vi "Connection Alive FGV A.vi"(0 "command":T2, 1 "IP address":string, 5 "connection ID":refnum<k5>, 9 "Name":string, 11 "error in (no error)":errorcluster, 12 "Message":string) -> (3 "Messages":string[](array[string]), 4 "Cluster":T1, 6 "Variant Out":variant, 8 "All connections":T1[](array[typedef]), 10 "all connections":refnum<k5>[](array[refnum]), 13 "Names":string[](array[string]), 14 "IP Addresses":string[](array[string]), 15 "error out":errorcluster)   [LabVIEW 2020]
uses:
  Connection Info.ctl
  Command.ctl
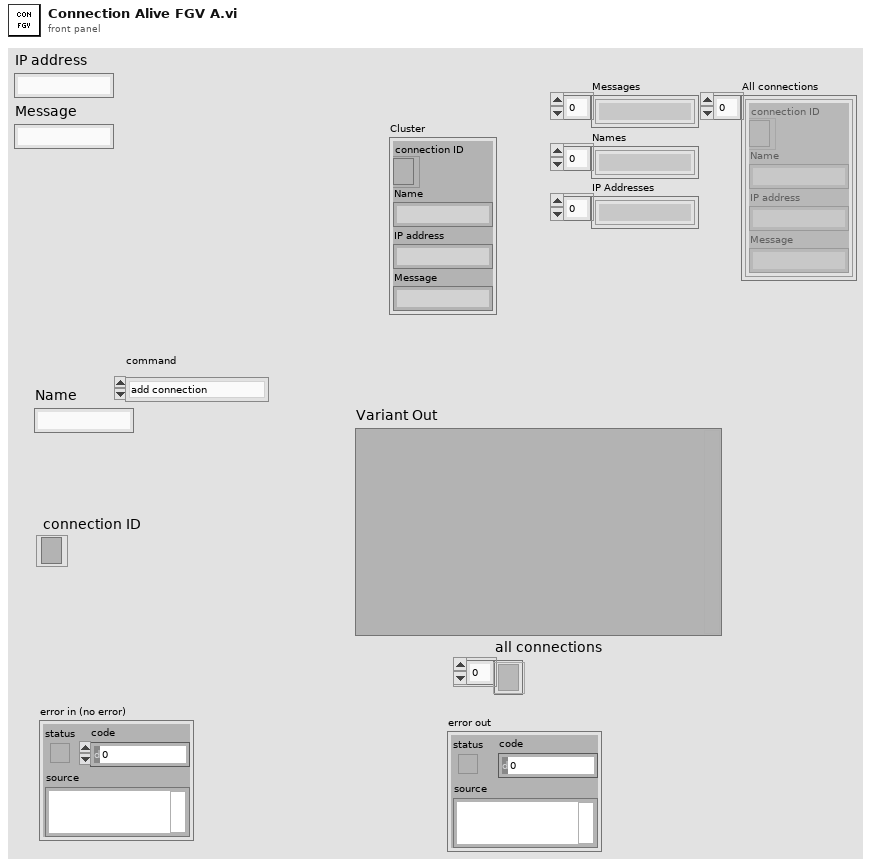
[diagram p1: front panel]
types:
  T1 = typedef "Connection Info.ctl" = cluster{"connection ID":refnum<k5>, "Name":string, "IP address":string, "Message":string}
  T2 = typedef "Command.ctl" = enum16{"add connection", "remove connection", "read connection data", "return all connections", "reset"}
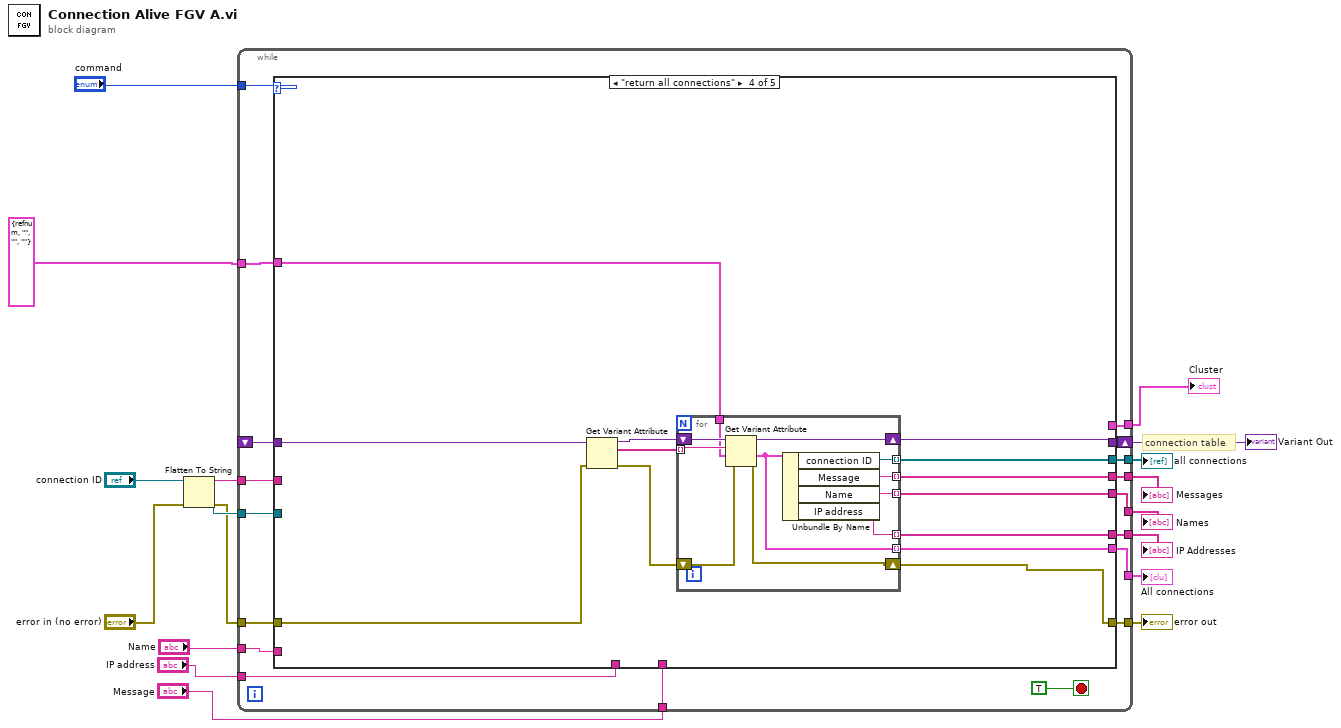
[diagram p0: block diagram]
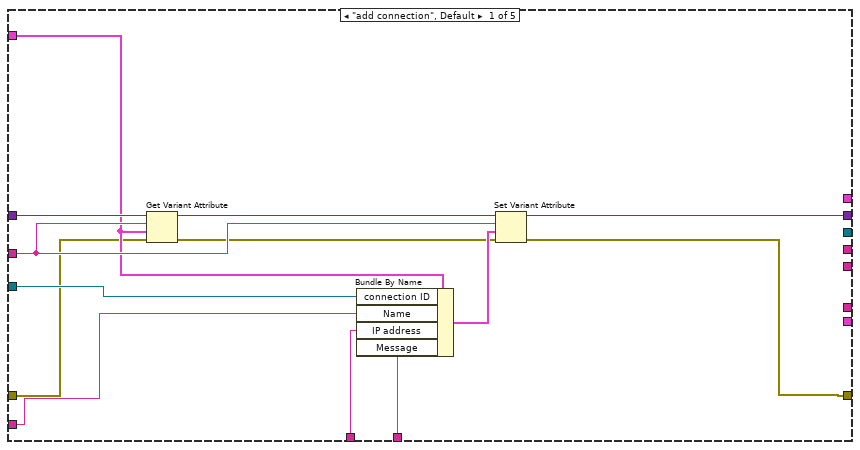
[diagram p2: hidden frame]
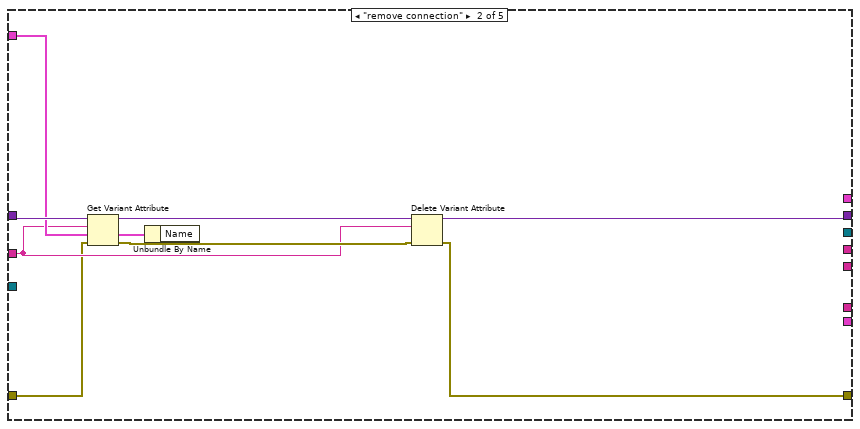
[diagram p3: hidden frame]
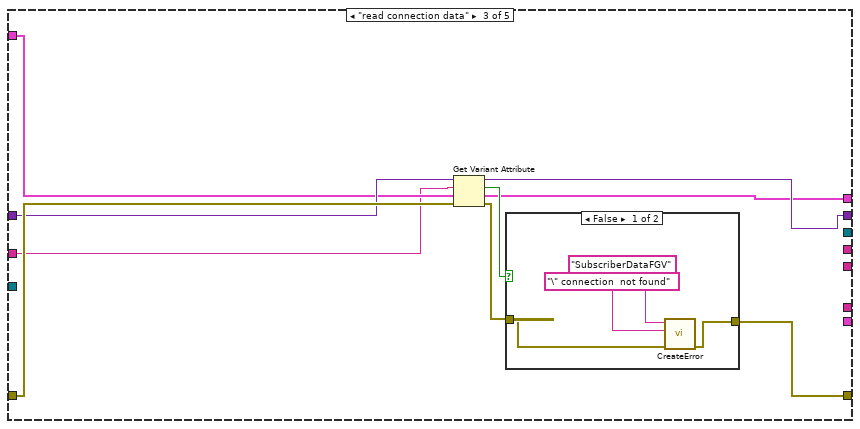
[diagram p4: hidden frame]
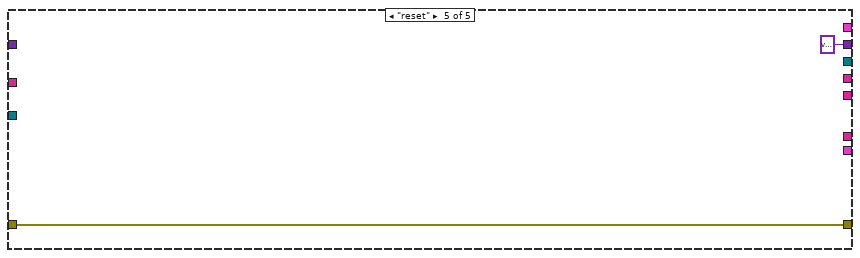
[diagram p6: hidden frame]
diagram:
  # "connection table"
  n1 = Flatten To String(anything="connection ID", error in (no error)="error in (no error)") -> (data string=w16:string, error out=w14:errorcluster)  [unwired: 2 in, 1 out]
  n2 = while {
    shift-right: [w35] -> w11
    shift-left: _ -> [w32]
    tunnel: "command" -> [w33]
    tunnel: "Name" -> [w31]
    tunnel: w16 -> [w30]
    tunnel: "connection ID" -> [w29]
    tunnel: T1 {"connection ID"=refnum, "Name"="", "IP address"="", "Message"=""} -> [w28]
    tunnel: w14 -> [w27]
    tunnel: [w26] -> w13
    tunnel: [w25] -> w8
    tunnel: [w24] -> w12
    tunnel: "IP address" -> [w23]
    tunnel: "Message" -> [w22]
    tunnel: [w21] -> w4
    tunnel: [w20] -> w3
    tunnel: [w19] -> w2
    tunnel: [w18] -> w1
    stop <- TRUE stop-if-true
    n3 = case shown="\"return all connections\"" w33 {
      tunnel: [w41 w51 w61 w81 variant ("Variant Out")] -> w35
      tunnel: w32 -> [w46 w57 w62 w84 _]
      tunnel: w31 -> [w38 _ _ _ _]
      tunnel: w30 -> [w44 w52 w59 _ _]
      tunnel: w29 -> [w47 _ _ _ _]
      tunnel: w28 -> [w43 w56 w60 w80 _]
      tunnel: w27 -> [w40 w50 w64 w78 w96]
      tunnel: [w39 w49 w63 w76 w96] -> w26
      tunnel: [_ _ w58 _ _] -> w25
      tunnel: [_ _ _ w79 _] -> w24
      tunnel: w23 -> [w37 _ _ _ _]
      tunnel: w22 -> [w36 _ _ _ _]
      tunnel: [_ _ _ w75 _] -> w21
      tunnel: [_ _ _ w74 _] -> w20
      tunnel: [_ _ _ w73 _] -> w19
      tunnel: [_ _ _ w72 _] -> w18
      frame "add connection", Default {
        n4 = Get Variant Attribute(Variant=w46, name=w44, default value (empty Variant)=w43, error in=w40) -> (duplicate Variant=w45:variant, error out=w42:errorcluster)  [unwired: 2 out]
        n5 = Bundle By Name(cluster=w43, "connection ID"=w47, "Name"=w38, "IP address"=w37, "Message"=w36) -> (w48:T1)
        n6 = Set Variant Attribute(Variant=w45, name=w44, value=w48, error in=w42) -> (Variant out=w41:variant, error out=w39:errorcluster)  [unwired: 1 out]
      }
      frame "remove connection" {
        n7 = Get Variant Attribute(Variant=w57, name=w52, default value (empty Variant)=w56, error in=w50) -> (duplicate Variant=w54:variant, value=w55:T1, error out=w53:errorcluster)  [unwired: 1 out]
        n8 = Unbundle By Name(w55) -> ()  [unwired: 1 out]
        n9 = Delete Variant Attribute(4:w53, 6:w52, 7:w54) -> (0:w49:errorcluster, 3:w51:variant)  [unwired: 1 out]
      }
      frame "read connection data" {
        n10 = Get Variant Attribute(Variant=w62, name=w59, default value (empty Variant)=w60, error in=w64) -> (duplicate Variant=w61:variant, found=w66:bool, value=w58:T1, error out=w65:errorcluster)
        n11 = case shown="False" w66 {
          tunnel: w65 -> [w69 w71]
          tunnel: [w68 w71] -> w63
          frame False {
            n12 = call "CreateError.vi"("user error in"=w69, "error message (\"\")"="\" connection  not found" ("error message (\"\")"), "command"="SubscriberDataFGV") -> ("user error  out"=w68:errorcluster)  [unwired: 8 in]
          }
          frame True {
          }
        }
      }
      frame "return all connections" {
        n13 = Get Variant Attribute(Variant=w84, error in=w78) -> (duplicate Variant=w82:variant, names=w83:string[], error out=w77:errorcluster)  [unwired: 2 in, 1 out]
        n14 = for {
          tunnel: w83 -> [w93] mode=indexing
          tunnel: w80 -> [w92]
          tunnel: [w91] -> w79 mode=indexing
          shift-right: [w94] -> w81
          shift-left: w82 -> [w95]
          shift-right: [w89] -> w76
          shift-left: w77 -> [w90]
          tunnel: [w88] -> w75 mode=indexing
          tunnel: [w87] -> w74 mode=indexing
          tunnel: [w86] -> w73 mode=indexing
          tunnel: [w85] -> w72 mode=indexing
          n15 = Get Variant Attribute(Variant=w95, name=w93, default value (empty Variant)=w92, error in=w90) -> (duplicate Variant=w94:variant, value=w85:T1, error out=w89:errorcluster)  [unwired: 1 out]
          n16 = Unbundle By Name(w85) -> ("connection ID"=w91:refnum<k5>, "Message"=w88:string, "Name"=w87:string, "IP address"=w86:string)
        }
      }
      frame "reset" {
      }
    }
  }
  "error out" <- w13
  "all connections" <- w12
  "Variant Out" <- w11
  "Cluster" <- w8
  "Messages" <- w4
  "Names" <- w3
  "IP Addresses" <- w2
  "All connections" <- w1
